vi "Global_CMD_SEN_Data In.vi"() -> ()   [LabVIEW 2023, in "PigeonIMU w Tilt_SEN.lvlib"]
uses:
  PigeonIMU w Tilt_SEN.lvlib
  Cluster_CMD_SEN_Data.ctl
panel:
  in  "CMD_SEN_Pigeon_Data":T1
  # "The Names of the Data items in the Global Variable MUST describe who the Single Writer is\nFor Command Globals the Commander(CMD) represents Teleop or Autonomous or other command loop.\nThe naming convention for a Command Sensor Global is:   \n\nCMD_SEN_SubSystem_Data Name\n\nExample:\nCMD_SEN_Gyro_Reset\nCMD_SEN_Distance_SetZero"
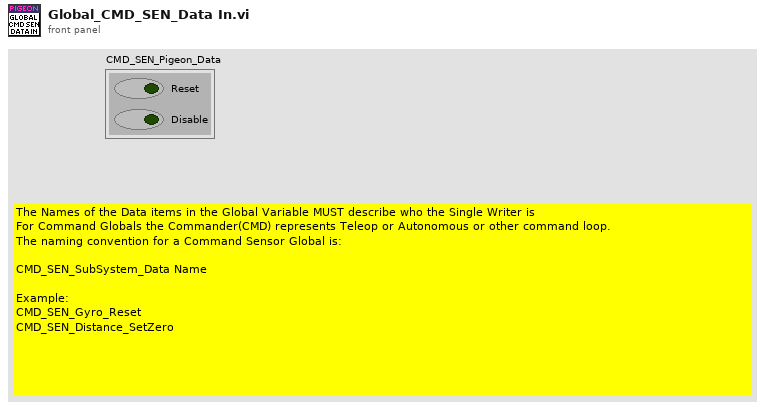
[diagram p1: front panel]
types:
  T1 = typedef "PigeonIMU w Tilt_SEN.lvlib/Cluster_CMD_SEN_Data.ctl" = cluster{"Reset":bool, "Disable":bool}
diagram:
